vi "Date to Dir Name (N.O.).vi"() -> (0 "Dir Name":string)   [LabVIEW 2009]
doc: "Creates a date string to use for creating a date-stamped directory, based on today's date."
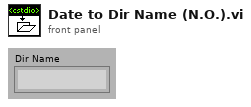
[diagram p1: front panel]
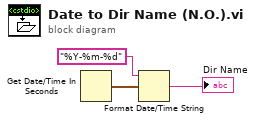
[diagram p0: block diagram]
diagram:
  n1 = Get Date/Time In Seconds() -> (seconds since 1Jan1904=w3:timestamp)
  n2 = Format Date/Time String(time format string (%c)="%Y-%m-%d", seconds (now)=w3) -> (date/time string=→"Dir Name":string)  [unwired: 1 out]
